vi "Destroy.vi"(8 "error in (no error)":errorcluster, 11 "CIF_UI in":refnum<class "CIF_UI.lvclass">) -> (0 "error out":errorcluster, 3 "CIF_UI out":refnum<class "CIF_UI.lvclass">)   [LabVIEW 2021, in "CIF_UI.lvclass"]
uses:
  CIF_UI.lvclass
  CIF_UI.lvclass/CIF_UI.ctl
  <vilib>/gRPC/LabVIEW gRPC Library/Shared/grpcId.ctl
  Instrument Studio/PluginSDK/Plugin Session.lvclass
  Typedef/Plugin Connection Map.ctl
  Typedef/Plugin Connections.ctl
  CIFPluginManager/CIFPluginManager/gRPC/CIF_Manager_client/RPC Messages/cif_manager_PluginInfo.ctl
  CIFPluginManager/CIFPluginManager/gRPC/CIF_Manager_client/RPC Messages/cif_manager_PluginVersion.ctl
  CIFPluginManager/CIFPluginManager/gRPC/CIF_Manager_client/RPC Messages/cif_plugincore_StatusData.ctl
  CIFPluginManager/CIFPluginManager/gRPC/CIF_Manager_client/RPC Messages/cif_plugincore_StatusData_State.ctl
  CIFPluginManager/CIFPluginManager/gRPC/CIF_Manager_client/RPC Messages/cif_plugincore_TimingStatistics.ctl
  CIFPluginManager/CIFPluginManager/gRPC/CIF_Manager_client/RPC Messages/cif_plugincore_TimingStatsBasic.ctl
  CIFPluginManager/CIFPluginManager/gRPC/CIF_Manager_client/RPC Messages/cif_plugincore_FifoStatistics.ctl
  CIFPluginManager/CIFPluginManager/gRPC/CIF_Manager_client/RPC Messages/cif_plugincore_Error.ctl
  CIFPluginManager/CIFPluginManager/gRPC/CIF_Manager_client/RPC Messages/cif_plugincore_MonitorDoubles.ctl
  CIFPluginManager/CIFPluginManager/gRPC/CIF_Manager_client/RPC Messages/cif_plugincore_MonitorU64.ctl
  CIFPluginManager/CIFPluginManager/gRPC/CIF_Manager_client/RPC Messages/cif_plugincore_MonitorI64.ctl
  CIFPluginManager/CIFPluginManager/gRPC/CIF_Manager_Client_Wrapper/CIFManagerClientWrapper.lvlib
  <vilib>/gRPC/LabVIEW gRPC Library/grpc-lvsupport-release.lvlib
  CIFPluginManager/CIFPluginManager/gRPC/CIF_Manager_client/CIF_Manager_client.lvlib
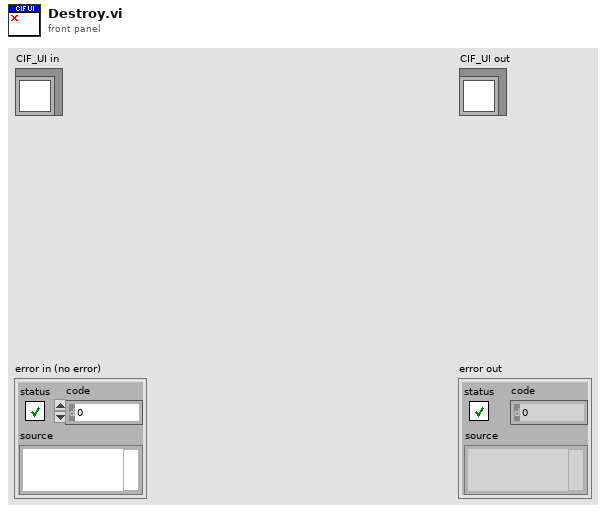
[diagram p1: front panel]
types:
  T1 = typedef "CIF_UI.lvclass/Plugin Connection Map.ctl" = map{string, T2}
  T2 = typedef "CIF_UI.lvclass/Plugin Connections.ctl" = cluster{"gRPC ID":T3, "Plugin info":T4}
  T3 = typedef "grpc-lvsupport-release.lvlib/grpcId.ctl" = u64
  T4 = typedef "CIF_Manager_client.lvlib/cif_manager_PluginInfo.ctl" = cluster{"plugin_name":string, "plugin_type":string, "grpc_port":i32, "plugin_version":T5, "status":T6}
  T5 = typedef "CIF_Manager_client.lvlib/cif_manager_PluginVersion.ctl" = cluster{"major_version":i32, "minor_version":i32, "fix_version":i32, "build_version":i32}
  T6 = typedef "CIF_Manager_client.lvlib/cif_plugincore_StatusData.ctl" = cluster{"state":T7, "timing_statistics":T8, "fifo_statistics":T10, "error":T11, "monitor_doubles":T12, "monitor_u64s":T13, "monitor_i64s":T14}
  T7 = typedef "CIF_Manager_client.lvlib/cif_plugincore_StatusData_State.ctl" = enum32{"NULL", "CREATING", "LISTENING", "RUNNING", "CLEANINGUP", "DESTROYING"}
  T8 = typedef "CIF_Manager_client.lvlib/cif_plugincore_TimingStatistics.ctl" = cluster{"period":T9, "wake_error":T9, "execute":T9, "housekeep":T9, "idle":T9}
  T9 = typedef "CIF_Manager_client.lvlib/cif_plugincore_TimingStatsBasic.ctl" = cluster{"max":i32, "min":i32}
  T10 = typedef "CIF_Manager_client.lvlib/cif_plugincore_FifoStatistics.ctl" = cluster{"from_t0":T9, "from_previous_plugin":T9, "output_error":T9}
  T11 = typedef "CIF_Manager_client.lvlib/cif_plugincore_Error.ctl" = cluster{"status":bool, "code":i32}
  T12 = typedef "CIF_Manager_client.lvlib/cif_plugincore_MonitorDoubles.ctl" = cluster{"double_1":dbl, "double_2":dbl, "double_3":dbl, "double_4":dbl}
  T13 = typedef "CIF_Manager_client.lvlib/cif_plugincore_MonitorU64.ctl" = cluster{"u64_1":u64, "u64_2":u64, "u64_3":u64, "u64_4":u64}
  T14 = typedef "CIF_Manager_client.lvlib/cif_plugincore_MonitorI64.ctl" = cluster{"i64_1":i64, "i64_2":i64, "i64_3":i64, "i64_4":i64}
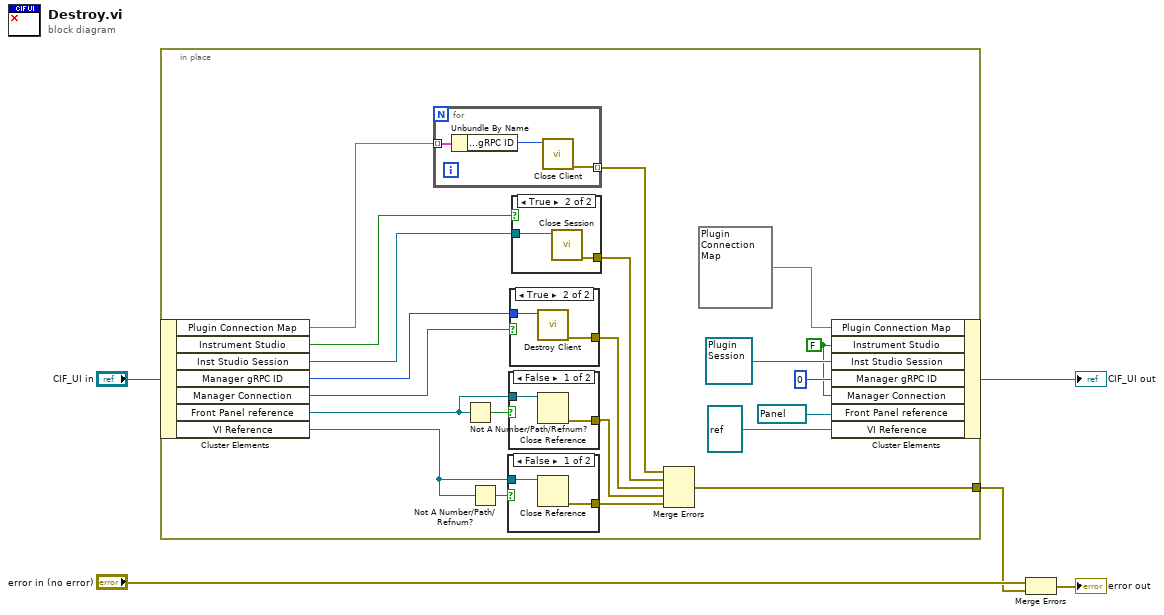
[diagram p0: block diagram]
diagram:
  n1 = in-place {
    in-place-border: [w15] -> w2
    w6 = FALSE ("Instrument Studio")
    n2 = in-place-cluster #1("CIF_UI in") -> ("Plugin Connection Map"=w10:T1, "Instrument Studio"=w14:bool, "Inst Studio Session"=w13:refnum<class "Plugin Session.lvclass">, "Manager gRPC ID"=w22:T3, "Manager Connection"=w7:bool, "Front Panel reference"=w23:refnum<vi>, "VI Reference"=w25:refnum<vi>)
    n3 = for {
      tunnel: w10 -> [w29] mode=indexing
      tunnel: [w27] -> w9 mode=indexing
      n4 = Unbundle By Name(w29) -> ("Plugin Connections.gRPC ID"=w28:T3)
      n5 = call <vilib>:"Close Client.vi"("ClientID in"=w28) -> ("error out"=w27:errorcluster)  [unwired: 10 in]
    }
    n6 = Not A Number/Path/Refnum?(number/path/refnum=w23) -> (NaN/Path/Refnum?=w24:bool)
    n7 = Not A Number/Path/Refnum?(number/path/refnum=w25) -> (NaN/Path/Refnum?=w26:bool)
    n8 = case shown="False" w26 {
      tunnel: w25 -> [w37 _]
      tunnel: [w36 _] -> w18
      frame False {
        n9 = Close Reference(reference=w37) -> (error out=w36:errorcluster)  [unwired: 1 in]
      }
      frame True {
      }
    }
    n10 = case shown="False" w24 {
      tunnel: w23 -> [w35 _]
      tunnel: [w34 _] -> w17
      frame False {
        n11 = Close Reference(reference=w35) -> (error out=w34:errorcluster)  [unwired: 1 in]
      }
      frame True {
      }
    }
    n12 = case shown="True" w7 {
      tunnel: w22 -> [_ w33]
      tunnel: [_ w32] -> w16
      frame False {
      }
      frame True {
        n13 = call "Destroy Client.vi"("gRPC ID"=w33) -> ("error out"=w32:errorcluster)  [unwired: 10 in]
      }
    }
    n14 = case shown="True" w14 {
      tunnel: w13 -> [_ w31]
      tunnel: [_ w30] -> w12
      frame False {
      }
      frame True {
        n15 = call "Close Session.vi"("Session in"=w31) -> ("error out"=w30:errorcluster)  [unwired: 10 in]
      }
    }
    n16 = Merge Errors(w9, w12, w16, w17, w18) -> (w15:errorcluster)
    n17 = in-place-cluster #1("Plugin Connection Map"=T1 {}, "Instrument Studio"=w6, "Inst Studio Session"=refnum<class "Plugin Session.lvclass"> refnum, "Manager gRPC ID"=T3 0 ("gRPC ID"), "Manager Connection"=w6, "Front Panel reference"=refnum<vi> refnum, "VI Reference"=refnum<vi> refnum) -> (→"CIF_UI out":refnum<class "CIF_UI.lvclass">)
  }
  n18 = Merge Errors("error in (no error)", w2) -> (→"error out":errorcluster)
